vi "StepperMotorOperate(SubVI).vi"(4 "DIR channel":u8, 5 "Photogate channel":u8, 6 "PUL channel":u8, 7 "ENA channel":u8, 8 "error in (no error)":errorcluster, 9 "Direction input":bool, 10 "Maximum steps\ninput":i32, 11 "LINX Resource in":T1) -> (0 "error out":errorcluster, 3 "LINX Resource out":T1)   [LabVIEW 2017]
uses:
  <vilib>/MakerHub/LINX/Private/Type Defs/LINX Ref.ctl
  <vilib>/MakerHub/LINX/Private/Type Defs/Platform.ctl
  <vilib>/MakerHub/LINX/Private/Type Defs/Interface.ctl
  <vilib>/MakerHub/LINX/Private/Device/Type Defs/LINX Device Config.ctl
  <vilib>/MakerHub/LINX/Private/Device/Type Defs/TCP Config.ctl
  <vilib>/MakerHub/LINX/Private/Device/Type Defs/Channels.ctl
  <vilib>/MakerHub/LINX/Public/Peripherals/Digital/Digital Write 1 Chan.vi
  <vilib>/MakerHub/LINX/Public/Peripherals/Analog/Analog Read 1 Chan.vi
  <vilib>/MakerHub/LINX/Public/Peripherals/Digital/Digital Write N Chans.vi
  <vilib>/MakerHub/LINX/Public/Peripherals/Analog/Analog Read N Chans.vi
  <vilib>/MakerHub/LINX/Private/Local IO/LinxDigitalWrite.vi
  <vilib>/MakerHub/LINX/Public/Utilities/Check Channel.vi
  <vilib>/MakerHub/LINX/Private/Local IO/LinxAnalogRead.vi
  <vilib>/MakerHub/LINX/Private/Utilties/Generate Error.vi
  <vilib>/MakerHub/LINX/LMH-LINX.lvlib
  <vilib>/MakerHub/LINX/Private/Device/Device.lvlib
panel:
  out "Voltage":dbl
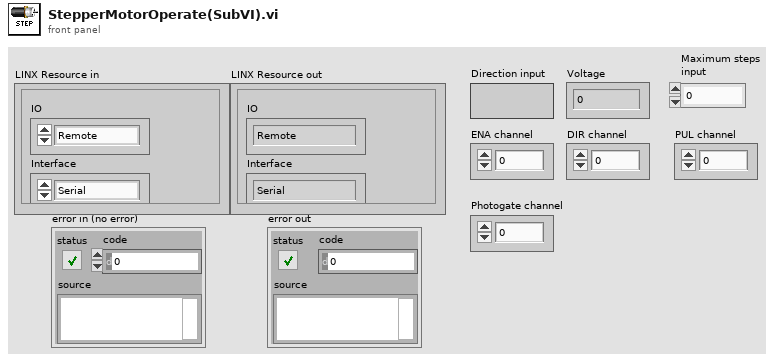
[diagram p1: front panel]
types:
  T1 = typedef "LMH-LINX.lvlib/LINX Ref.ctl" = cluster{"IO":T2, "Interface":T3, "LINX Device Config":T4}
  T2 = typedef "LMH-LINX.lvlib/Platform.ctl" = enum16{"Remote", "Local"}
  T3 = typedef "LMH-LINX.lvlib/Interface.ctl" = enum16{"Serial", "TCP"}
  T4 = typedef "LMH-LINX.lvlib/Device.lvlib/LINX Device Config.ctl" = cluster{"Interface":T3, "COM Port":refnum<visa-resource-name>, "TCP Configuration":T5, "Device Family":u8, "Device ID":u8, "Device Name":string, "TCP Ref":refnum<k5>, "Channels":T6}
  T5 = typedef "LMH-LINX.lvlib/Device.lvlib/TCP Config.ctl" = cluster{"IP Address":string, "Port":u16}
  T6 = typedef "LMH-LINX.lvlib/Channels.ctl" = cluster{"DI":u8[], "DO":u8[], "AI":u8[], "AO":u8[], "PWM":u8[], "QE":u8[], "UART":u8[], "I2C 2":u8[], "SPI":u8[], "CAN":u8[], "Servo":u8[], "AI Ref (V)":dbl, "AI Resolution (Bits)":u8, "AO Ref (V)":dbl, "AO Resolution (Bits)":u8}
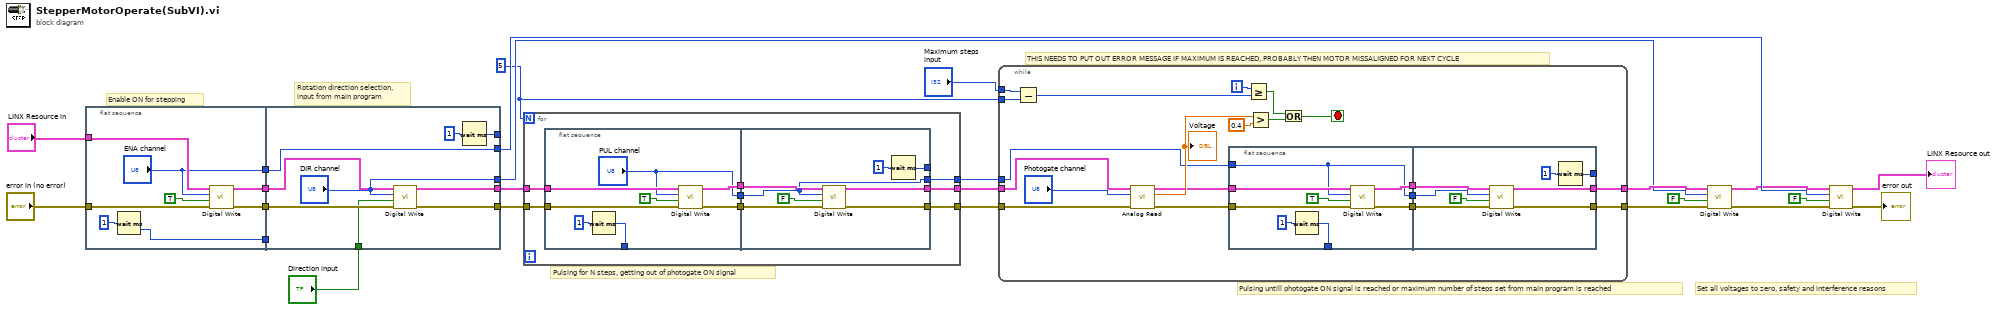
[diagram p0: block diagram]
diagram:
  w1 = 5
  # "Set all voltages to zero, safety and interference reasons"
  # "THIS NEEDS TO PUT OUT ERROR MESSAGE IF MAXIMUM IS REACHED, PROBABLY THEN MOTOR MISSALIGNED FOR NEXT CYCLE"
  # "Pulsing untill photogate ON signal is reached or maximum number of steps set from main program is reached"
  # "Pulsing for N steps, getting out of photogate ON signal"
  # "Rotation direction selection,\ninput from main program"
  # "Enable ON for stepping"
  n1 = flat-sequence {
    tunnel: [w31] -> w24
    tunnel: "LINX Resource in" -> [w30]
    tunnel: [w29] -> w22
    tunnel: "error in (no error)" -> [w28]
    tunnel: [w27] -> w20
    tunnel: ["ENA channel"] -> w10
    tunnel: [w40] -> _
    tunnel: w24 -> [_]
    tunnel: w22 -> [w39]
    tunnel: [w38] -> w19
    tunnel: w20 -> [w37]
    tunnel: [w36] -> w17
    tunnel: "Direction input" -> [w35]
    tunnel: [w34] -> w11
    tunnel: w10 -> [w34]
    tunnel: ["DIR channel"] -> w3
    frame #0 {
      n2 = Wait (ms)(milliseconds to wait=u32 1) -> (millisecond timer value=w31:u32)
      n3 = call-poly <vilib>:"Digital Write.vi"("Error In"=w28, "Output Value"=TRUE, "DO Channel"="ENA channel", "LINX Resource"=w30) -> ("Error Out"=w27:errorcluster, "LINX Resource"=w29:T1)  [unwired: 6 in]
    }
    frame #1 {
      n4 = call-poly <vilib>:"Digital Write.vi"("Error In"=w37, "Output Value"=w35, "DO Channel"="DIR channel", "LINX Resource"=w39) -> ("Error Out"=w36:errorcluster, "LINX Resource"=w38:T1)  [unwired: 6 in]
      n5 = Wait (ms)(milliseconds to wait=u32 1) -> (millisecond timer value=w40:u32)
    }
  }
  n6 = for {
    N: w1 -> [_]
    tunnel: w19 -> [w49]
    tunnel: [w48] -> w18
    tunnel: w17 -> [w47]
    tunnel: [w46] -> w16
    tunnel: [w42] -> w9
    n7 = flat-sequence {
      tunnel: [w56] -> _
      tunnel: w49 -> [w55]
      tunnel: w47 -> [w54]
      tunnel: [w53] -> w45
      tunnel: [w52] -> w44
      tunnel: ["PUL channel"] -> w43
      tunnel: [w64] -> _
      tunnel: [w60] -> w48
      tunnel: [w62] -> w46
      tunnel: w45 -> [w63]
      tunnel: w44 -> [w61]
      tunnel: w43 -> [w58]
      tunnel: [w58] -> w42
      frame #0 {
        n8 = Wait (ms)(milliseconds to wait=u32 1) -> (millisecond timer value=w56:u32)
        n9 = call-poly <vilib>:"Digital Write.vi"("Error In"=w54, "Output Value"=TRUE, "DO Channel"="PUL channel", "LINX Resource"=w55) -> ("Error Out"=w53:errorcluster, "LINX Resource"=w52:T1)  [unwired: 6 in]
      }
      frame #1 {
        n10 = call-poly <vilib>:"Digital Write.vi"("Error In"=w63, "Output Value"=FALSE, "DO Channel"=w58, "LINX Resource"=w61) -> ("Error Out"=w62:errorcluster, "LINX Resource"=w60:T1)  [unwired: 6 in]
        n11 = Wait (ms)(milliseconds to wait=u32 1) -> (millisecond timer value=w64:u32)
      }
    }
  }
  n12 = while {
    tunnel: [w79] -> w8
    tunnel: w16 -> [w81]
    tunnel: [w78] -> w5
    tunnel: w18 -> [w76]
    tunnel: w9 -> [w73]
    tunnel: "Maximum steps\ninput" -> [w68]
    tunnel: w1 -> [w67]
    i -> [w69]
    stop <- w71 stop-if-true
    n13 = Subtract(x=w68, y=w67) -> (x-y=w66:i32)
    n14 = call-poly <vilib>:"Analog Read.vi"("Error In"=w81, "Analog Channel"="Photogate channel", "LINX Resource"=w76) -> ("Error Out"=w82:errorcluster, "Voltage"=w85:dbl, "LINX Resource"=w83:T1)  [unwired: 5 in, 1 out]
    "Voltage" <- w85
    n15 = flat-sequence {
      tunnel: w83 -> [w91]
      tunnel: w82 -> [w90]
      tunnel: w73 -> [w87]
      tunnel: [w87] -> w77
      tunnel: [w92] -> _
      tunnel: [w89] -> w75
      tunnel: [w88] -> w74
      tunnel: [w95] -> w79
      tunnel: [w94] -> w78
      tunnel: w77 -> [w97]
      tunnel: [w100] -> _
      tunnel: w75 -> [w99]
      tunnel: w74 -> [w98]
      frame #0 {
        n16 = Wait (ms)(milliseconds to wait=u32 1) -> (millisecond timer value=w92:u32)
        n17 = call-poly <vilib>:"Digital Write.vi"("Error In"=w90, "Output Value"=TRUE, "DO Channel"=w87, "LINX Resource"=w91) -> ("Error Out"=w89:errorcluster, "LINX Resource"=w88:T1)  [unwired: 6 in]
      }
      frame #1 {
        n18 = call-poly <vilib>:"Digital Write.vi"("Error In"=w99, "Output Value"=FALSE, "DO Channel"=w97, "LINX Resource"=w98) -> ("Error Out"=w94:errorcluster, "LINX Resource"=w95:T1)  [unwired: 6 in]
        n19 = Wait (ms)(milliseconds to wait=u32 1) -> (millisecond timer value=w100:u32)
      }
    }
    n20 = Greater Or Equal?(x=w69, y=w66) -> (x >= y?=w70:bool)
    n21 = Greater?(x=w85, y=0.4) -> (0:w72:bool)
    n22 = Or(x=w70, y=w72) -> (x .or. y?=w71:bool)
  }
  n23 = call-poly <vilib>:"Digital Write.vi"("Error In"=w5, "Output Value"=FALSE, "DO Channel"=w3, "LINX Resource"=w8) -> ("Error Out"=w6:errorcluster, "LINX Resource"=w7:T1)  [unwired: 6 in]
  n24 = call-poly <vilib>:"Digital Write.vi"("Error In"=w6, "Output Value"=FALSE, "DO Channel"=w11, "LINX Resource"=w7) -> ("Error Out"=→"error out":errorcluster, "LINX Resource"=→"LINX Resource out":T1)  [unwired: 6 in]
